vi "Init 5782.vi"(4 "User Data 1":u8=64, 6 "Record length":u16, 7 "Use 1Mhz clock":bool, 8 "error in (no error)":errorcluster, 9 "Mode":T3, 10 "Clock Source":T2(ring), 11 "FPGA ref":T1) -> (0 "error out":errorcluster, 3 "FpgaRef5782 Out":refnum<class "FpgaRef5782.lvclass">)   [LabVIEW 2013, in "FpgaRef5782.lvclass"]
uses:
  FpgaRef5782.lvclass
  FPGA/DataMode.ctl
  5782 FPGA ref.ctl
  FPGA/fpga_settings.ctl
  FpgaRef5782.lvclass/FpgaRef5782.ctl
  <vilib>/rvi/interface/common/niFpgaWaitOnOcc.vi
  <vilib>/Utility/error.llb/Error Cluster From Error Code.vi
  <vilib>/rvi/errors/niLvFpgaAdjustHostInterfaceError.vi
  <vilib>/rvi/interface/nirviReadWriteControl/nirviReadWriteControl.xnode
  NiFpgaLv.dll
  <vilib>/rvi/interface/Simulation/niFpgaSimulationCallBeginRW.vi
  FpgaRefBase/FpgaRefBase.lvclass
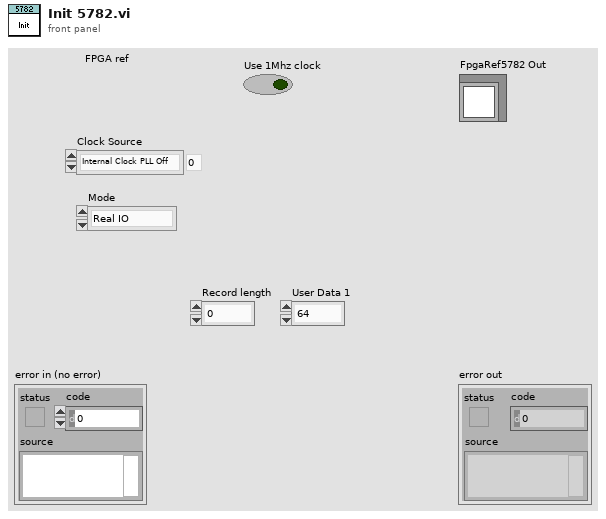
[diagram p1: front panel]
types:
  T1 = typedef "5782 FPGA ref.ctl" = refnum<k20>
  T2 = enum8{"Internal Clock PLL Off", "Internal Clock PLL On (REF IN)", "External Clock (CLK_IN)", "Internal Clock PLL On (IoModSyncClk)"}
  T3 = typedef "DataMode.ctl" = enum16{"Real IO", "Simulated"}
  T4 = typedef "fpga_settings.ctl" = enum16{"Feedback Enable", "New FIR coeffs", "FIR shift", "Enable filter", "Set Downsample", "Downsample", "CIC Gain", "Record length", "Trigger samples", "Quiet time", "a_am", "b_am", "Use fixed delay", "fixed sin_fi", "fixed cos_fi", "Ki*Tau", "Kp", "Kd_Tau", "Fi_start", "Fi_delta", "DC_offs 0", "DC_offs 1", "DC_offs 2", "DC_offs 3", "Ki*Tau am", "Kp am", "Kd_Tau am", "Feedback AM"}
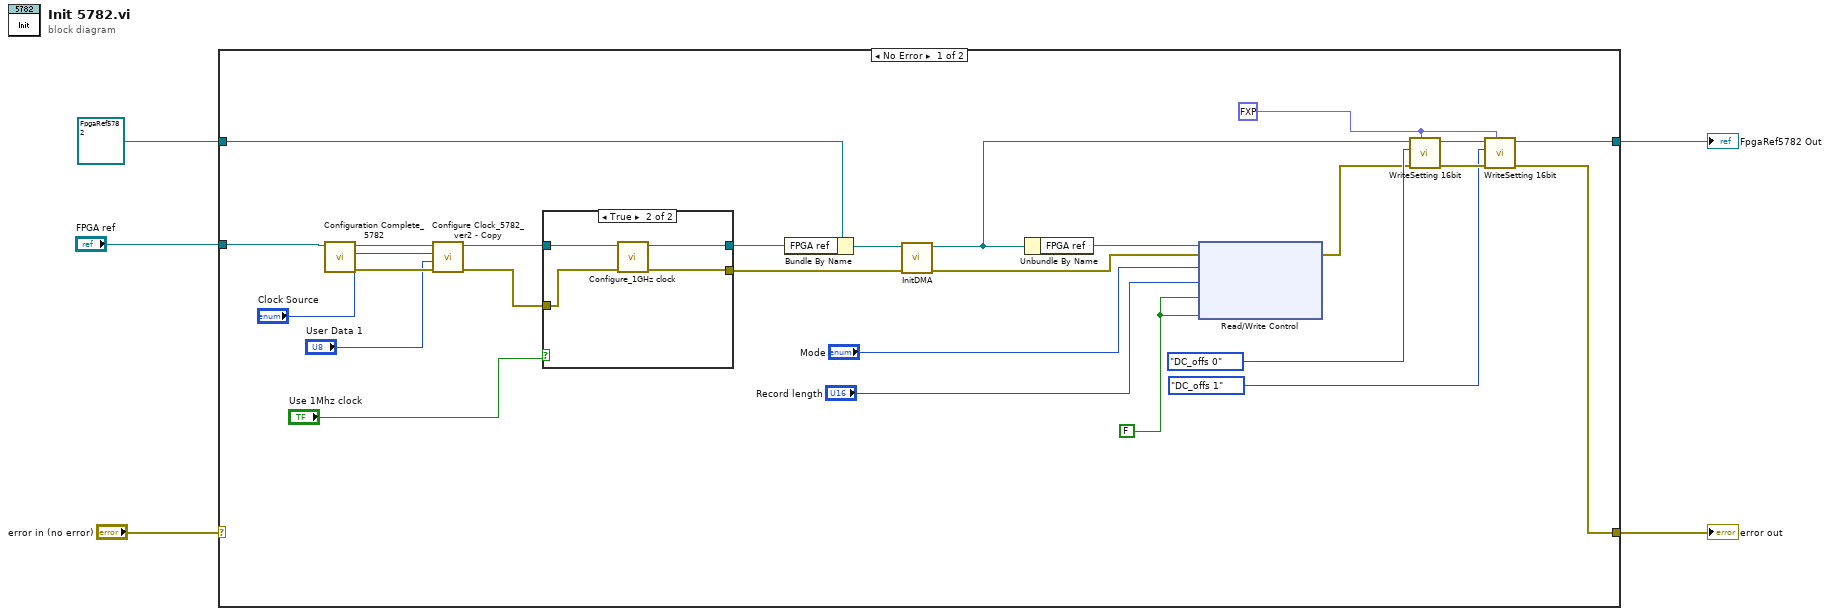
[diagram p0: block diagram]
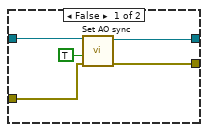
[diagram p2: hidden frame]
diagram:
  n1 = case shown="No Error" "error in (no error)" {
    selector: "error in (no error)" -> [_ w42]
    tunnel: [w8 w42] -> w4
    tunnel: [w12 w41] -> w3
    tunnel: refnum<class "FpgaRef5782.lvclass"> refnum ("FpgaRef5782 Out") -> [w30 w41]
    tunnel: "FPGA ref" -> [w18 _]
    frame No Error {
      w14 = fxp<+,16,16> 0.0 ("value")
      w29 = FALSE
      n2 = call "Configuration Complete_5782.vi"("FPGA VI Reference in"=w18) -> ("error out"=w24:errorcluster, "FPGA VI Reference out"=w23:T1)  [unwired: 8 in, 1 out]
      n3 = call "Configure Clock_5782_ver2 - Copy.vi"("error in"=w24, "User Data 1"="User Data 1", "Clock Source"="Clock Source", "FPGA VI Reference"=w23) -> ("error out"=w7:errorcluster, "FPGA VI Reference out"=w19:T1)  [unwired: 5 in, 1 out]
      n4 = case shown="True" "Use 1Mhz clock" {
        tunnel: [w34 w40] -> w20
        tunnel: w19 -> [w35 w39]
        tunnel: w7 -> [w33 w38]
        tunnel: [w32 w37] -> w6
        frame False {
          n5 = call "Set AO sync.vi"("error in"=w33, "AO sync"=TRUE, "FPGA SPI config ref"=w35) -> ("error out"=w32:errorcluster, "FPGA SPI config out"=w34:T1)  [unwired: 7 in]
        }
        frame True {
          n6 = call "Configure_1GHz clock.vi"("error in"=w38, "FPGA SPI config ref"=w39) -> ("error out"=w37:errorcluster, "FPGA SPI config out"=w40:T1)  [unwired: 8 in]
        }
      }
      n7 = Bundle By Name(cluster=w30, "FPGA ref"=w20) -> (w31:refnum<class "FpgaRef5782.lvclass">)
      n8 = call-dynamic "InitDMA.vi"("error in (no error)"=w6, "FpgaRef5782 in"=w31) -> ("error out"=w17:errorcluster, "FpgaRef5782 out"=w13:refnum<class "FpgaRef5782.lvclass">)  [unwired: 8 in]
      n9 = Unbundle By Name(w13) -> ("FPGA ref"=w28:T1)
      n10 = xnode "Read/Write Control"("FPGA VI Reference In"=w28, "error in"=w17, "Mode"="Mode", "5782 record length"="Record length", "Trigger Acquisition"=w29, "Acquisition running"=w29) -> ("error out"=w9:errorcluster)  [unwired: 1 out]
      n11 = call "WriteSetting 16bit.vi"("value"=w14, "error in (no error)"=w9, "FPGA Setting"=fpga_settings."DC_offs 0", "FpgaRefBase in"=w13) -> ("error out"=w15:errorcluster, "FpgaRefBase out"=w16:refnum<class "FpgaRef5782.lvclass">)  [unwired: 6 in]
      n12 = call "WriteSetting 16bit.vi"("value"=w14, "error in (no error)"=w15, "FPGA Setting"=fpga_settings."DC_offs 1", "FpgaRefBase in"=w16) -> ("error out"=w8:errorcluster, "FpgaRefBase out"=w12:refnum<class "FpgaRef5782.lvclass">)  [unwired: 6 in]
    }
    frame Error {
    }
  }
  "error out" <- w4
  "FpgaRef5782 Out" <- w3
